vi "Are Equal.vi"(8 "error in":errorcluster, 9 "Recieved File Path":path, 10 "Approved File Path":path, 11 "File Comparator in":refnum<class "File Comparator.lvclass">) -> (0 "error out":errorcluster, 2 "Are Equal?":bool, 3 "File Comparator out":refnum<class "File Comparator.lvclass">)   [LabVIEW 2020, in "Approval Tests.lvlib" / "File Comparator.lvclass"]
uses:
  File Comparator.lvclass
  <vilib>/security/Message Digest/API/Instances/File/SHA-256 File Checksum.vi
  <vilib>/security/Message Digest/API/NI_Message Digest API.lvlib
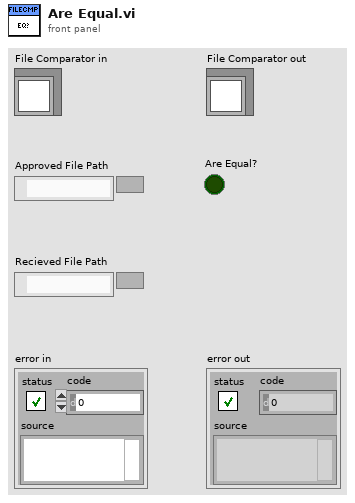
[diagram p1: front panel]
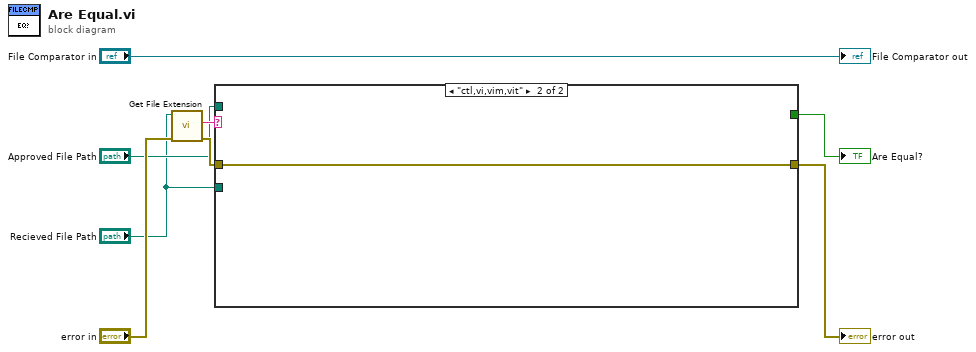
[diagram p0: block diagram]
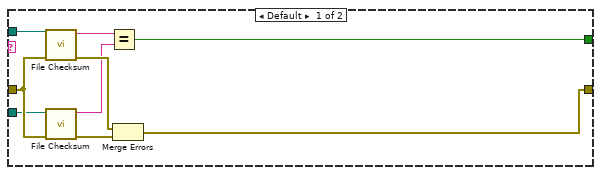
[diagram p2: hidden frame]
diagram:
  n1 = call <vilib>:"Get File Extension.vi"("error in (no error)"="error in", "file"="Recieved File Path") -> ("error out"=w8:errorcluster, "lowercase file extension"=w4:string)  [unwired: 5 in, 3 out]
  n2 = case shown="\"ctl,vi,vim,vit\"" w4 {
    tunnel: [w14 w18] -> w6
    tunnel: [w9 _] -> w1
    tunnel: w8 -> [w17 w18]
    tunnel: "Approved File Path" -> [w13 _]
    tunnel: "Recieved File Path" -> [w12 _]
    frame Default {
      n3 = call-poly <vilib>:"File Checksum.vi"("error in"=w17, "path"=w13) -> ("error out"=w15:errorcluster, "digest"=w11:string)  [unwired: 8 in]
      n4 = call-poly <vilib>:"File Checksum.vi"("error in"=w17, "path"=w12) -> ("error out"=w16:errorcluster, "digest"=w10:string)  [unwired: 8 in]
      n5 = Equal?(x=w11, y=w10) -> (x = y?=w9:bool)
      n6 = Merge Errors(w15, w16) -> (w14:errorcluster)
    }
    frame "ctl,vi,vim,vit" {
    }
  }
  "error out" <- w6
  "Are Equal?" <- w1
  "File Comparator out" <- "File Comparator in"
